vi "PitchRoll.vi"() -> ()   [LabVIEW 2016]
uses:
  <vilib>/MakerHub/LINX/Private/Type Defs/Interface.ctl
  <vilib>/MakerHub/LINX/Public/Sensors/Accelerometer/MPU60X0/DeviceAddresses.ctl
  <vilib>/MakerHub/LINX/LMH-LINX.lvlib
  <vilib>/MakerHub/LINX/Public/Sensors/Accelerometer/MPU60X0/MPU60X0.lvlib
panel:
  out "come":bool
  out "help":bool
  out "Pitch":dbl
  out "Roll":dbl
  out "Acceleration Data":T1
  in  "STOP":bool
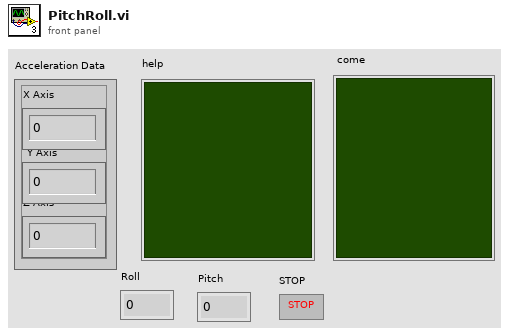
[diagram p1: front panel]
types:
  T1 = cluster{"X Axis":i16, "Y Axis":i16, "Z Axis":i16}
  T2 = typedef "LMH-LINX.lvlib/MPU60X0.lvlib/DeviceAddresses.ctl" = enum16{"0x68", "0x69"}
  T3 = typedef "LMH-LINX.lvlib/Interface.ctl" = enum16{"Serial", "TCP"}
  T4 = typedef "LMH-LINX.lvlib/LINX Ref.ctl" = cluster{"Platform":T5, "Interface":T3, "LINX Device Config":T6}
  T5 = typedef "LMH-LINX.lvlib/Platform.ctl" = enum16{"LINX", "myRIO"}
  T6 = typedef "LMH-LINX.lvlib/Device.lvlib/LINX Device Config.ctl" = cluster{"Interface":T3, "COM Port":refnum<visa-resource-name>, "TCP Configuration":T7, "Device Family":u8, "Device ID":u8, "Device Name":string, "TCP Ref":refnum<k5>, "Channels":T8}
  T7 = typedef "LMH-LINX.lvlib/Device.lvlib/TCP Config.ctl" = cluster{"IP Address":string, "Port":u16}
  T8 = typedef "LMH-LINX.lvlib/Channels.ctl" = cluster{"DI":u8[], "DO":u8[], "AI":u8[], "AO":u8[], "PWM":u8[], "QE":u8[], "UART":u8[], "I2C 2":u8[], "SPI":u8[], "CAN":u8[], "Servo":u8[], "AI Ref (V)":dbl, "AO Ref (V)":dbl, "AO Resolution (Bits)":u8}
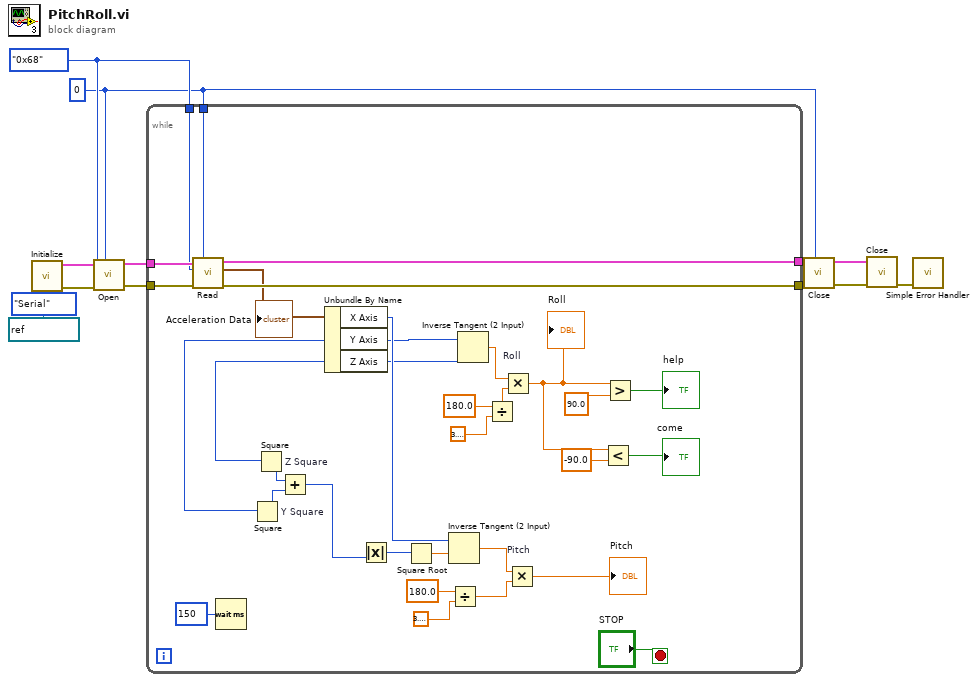
[diagram p0: block diagram]
diagram:
  w2 = u8 0 ("I2C Channel")
  w3 = DeviceAddresses."0x68" ("Device Address")
  n1 = call <vilib>:"Initialize.vi"("Serial Port"=refnum<visa-resource-name> "COM3", "Interface"=Interface."Serial") -> ("Error Out"=w6:errorcluster, "LINX Ref"=w13:T4)  [unwired: 7 in, 1 out]
  n2 = call <vilib>:"Open.vi"("I2C Channel"=w2, "Error In"=w6, "Device Address"=w3, "LINX Resource"=w13) -> ("Error Out"=w7:errorcluster, "LINX Resource"=w12:T4)  [unwired: 6 in]
  n3 = while {
    tunnel: w12 -> [w44]
    tunnel: [w43] -> w11
    tunnel: [w42] -> w8
    tunnel: w7 -> [w41]
    tunnel: w3 -> [w40]
    tunnel: w2 -> [w39]
    stop <- "STOP" stop-if-true
    n4 = call <vilib>:"Read.vi"("I2C Channel"=w39, "Error In"=w41, "Device Address"=w40, "LINX Resource"=w44) -> ("Error Out"=w42:errorcluster, "Acceleration Data"=w36:T1, "LINX Resource"=w43:T4)  [unwired: 3 in, 2 out]
    "Acceleration Data" <- w36
    n5 = Wait (ms)(milliseconds to wait=u32 150) -> ()  [unwired: 1 out]
    n6 = Unbundle By Name(w36) -> ("X Axis"=w31:i16, "Y Axis"=w30:i16, "Z Axis"=w29:i16)
    n7 = Square "Y Square"(x=w30) -> (x^2=w28:i16)
    n8 = Square "Z Square"(x=w29) -> (x^2=w27:i16)
    n9 = Add(x=w27, y=w28) -> (x+y=w20:i16)
    n10 = Absolute Value(x=w20) -> (abs(x)=w21:i16)
    n11 = Square Root(x=w21) -> (sqrt(x)=w19:dbl)
    n12 = Inverse Tangent (2 Input)(1:w19, 2:w31) -> (0:w22:dbl)
    n13 = Divide(x=180.0, y=3.141592653589793) -> (x/y=w23:dbl)
    n14 = Inverse Tangent (2 Input)(1:w29, 2:w30) -> (0:w35:dbl)
    n15 = Divide(x=180.0, y=3.141592653589793) -> (x/y=w32:dbl)
    n16 = Multiply "Roll"(x=w35, y=w32) -> (x*y=w16:dbl)
    "Roll" <- w16
    n17 = Multiply "Pitch"(x=w22, y=w23) -> (x*y=→"Pitch":dbl)
    n18 = Less?(x=w16, y=-90.0) -> (x < y?=→"come":bool)
    n19 = Greater?(x=w16, y=90.0) -> (0:→"help":bool)
  }
  n20 = call <vilib>:"Close.vi"("I2C Channel"=w2, "Error In"=w8, "LINX Resource"=w11) -> ("Error Out"=w9:errorcluster, "LINX Resource"=w10:T4)  [unwired: 7 in]
  n21 = call <vilib>:"Close.vi"("Error In"=w9, "LINX Resource"=w10) -> ("Error Out"=w1:errorcluster)  [unwired: 8 in, 1 out]
  n22 = call <vilib>:"Simple Error Handler.vi"("error in (no error)"=w1) -> ()  [unwired: 4 in, 5 out]
